vi "Visual Map.vi"() -> ()   [LabVIEW 2015, in "Circle the Wagons.lvclass"]
uses:
  Circle the Wagons.lvclass
panel:
  out "Array":bool[][](array[boolean])=[[TRUE, TRUE, TRUE, TRUE, TRUE, TRUE, TRUE, TRUE, FALSE], [TRUE, FALSE, FALSE, FALSE, FALSE, FALSE, FALSE, TRUE, FALSE], [TRUE, FALSE, TRUE, FALSE, TRUE, FALSE, FALSE, TRUE, FALSE], [TRUE, FALSE, FALSE, FALSE, FALSE, TRUE, FALSE, TRUE, FALSE], [TRUE, FALSE, TRUE, FALSE, FALSE, FALSE, FALSE, TRUE, FALSE], [TRUE, FALSE, FALSE, TRUE, FALSE, TRUE, FALSE, TRUE, FALSE], [TRUE, FALSE, FALSE, FALSE, FALSE, FALSE, FALSE, TRUE, FALSE], [TRUE, TRUE, TRUE, TRUE, TRUE, TRUE, TRUE, TRUE, FALSE], [FALSE, FALSE, FALSE, FALSE, FALSE, FALSE, FALSE, FALSE, FALSE]]
  # "0   1   2   3   4   5   6   7   8   9"
  # "0\n1\n2\n3\n4\n5\n6\n7\n8\n9"
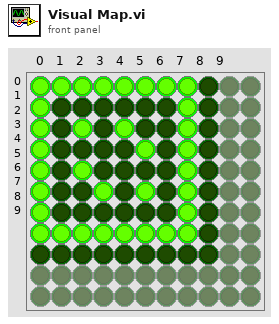
[diagram p1: front panel]
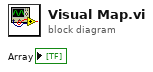
[diagram p0: block diagram]
diagram:
